vi "extractModuleContents.vi"(8 "error in (no error)":errorcluster, 11 "IDLFile in":refnum<class "IDLFile.lvclass">) -> (0 "error out":errorcluster, 2 "moduleContentsString":string, 3 "IDLFile out":refnum<class "IDLFile.lvclass">)   [LabVIEW 2016, in "IDLFile.lvclass"]
uses:
  IDLFile.lvclass
  IDLFile.lvclass/IDLFile.ctl
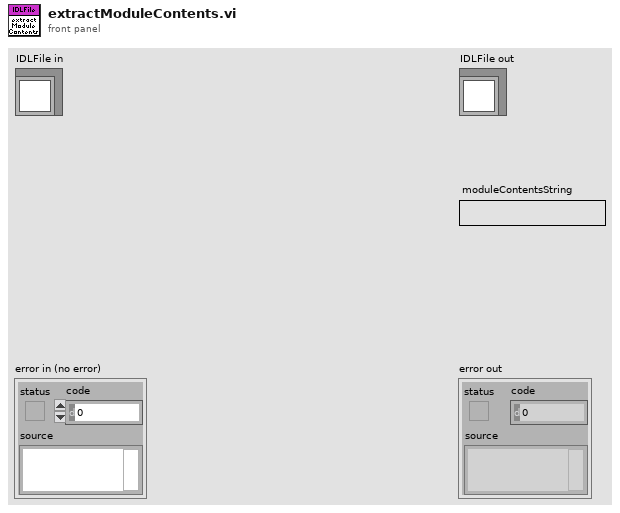
[diagram p1: front panel]
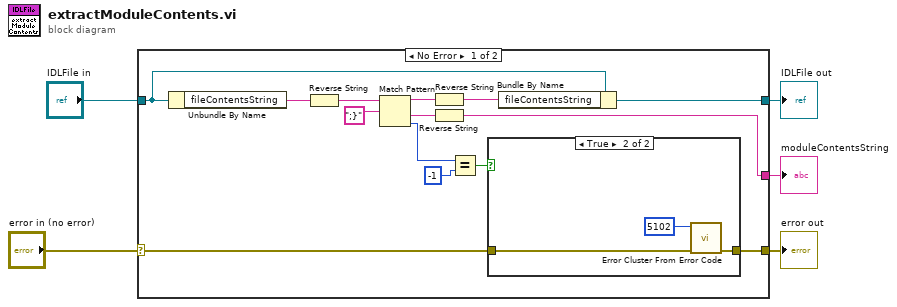
[diagram p0: block diagram]
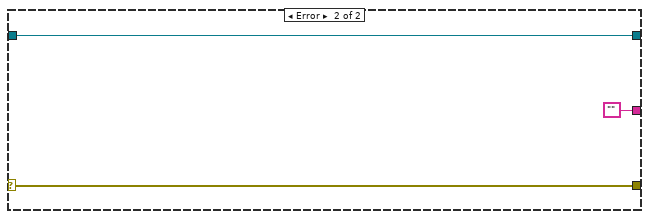
[diagram p3: hidden frame]
diagram:
  n1 = case shown="No Error" "error in (no error)" {
    selector: "error in (no error)" -> [w10 w26]
    tunnel: [w9 w26] -> w4
    tunnel: [w12 w25] -> w2
    tunnel: "IDLFile in" -> [w13 w25]
    tunnel: [w11 ""] -> w1
    frame No Error {
      n2 = Unbundle By Name(w13) -> ("fileContentsString"=w14:string)
      n3 = Reverse String(1:w14) -> (0:w19:string)
      n4 = Match Pattern(string=w19, regular expression=";}") -> (before substring=w7:string, after substring=w18:string, offset past match=w16:i32)  [unwired: 1 in, 1 out]
      n5 = Reverse String(1:w7) -> (0:w6:string)
      n6 = Reverse String(1:w18) -> (0:w11:string)
      n7 = Equal?(x=w16, y=-1) -> (x = y?=w8:bool)
      n8 = case shown="True" w8 {
        tunnel: w10 -> [w20 w22]
        tunnel: [w20 w21] -> w9
        frame False {
        }
        frame True {
          n9 = call <vilib>:"Error Cluster From Error Code.vi"("error in (no error)"=w22, "error code (0)"=5102) -> ("error out"=w21:errorcluster)  [unwired: 7 in]
        }
      }
      n10 = Bundle By Name(cluster=w13, "fileContentsString"=w6) -> (w12:refnum<class "IDLFile.lvclass">)
    }
    frame Error {
    }
  }
  "error out" <- w4
  "IDLFile out" <- w2
  "moduleContentsString" <- w1
